vi "String1-2 to OK-NG.vi"(11 "String":string) -> (3 "String Out":string)   [LabVIEW 2021]
doc: "input 1: = OK\ninput 2: = NG\nother \ninput = ouput"
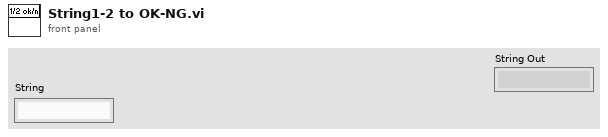
[diagram p1: front panel]
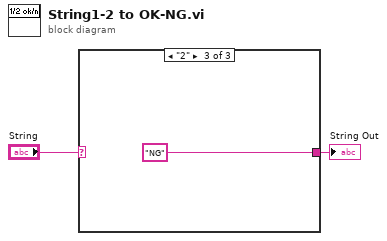
[diagram p0: block diagram]
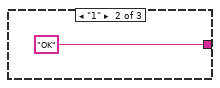
[diagram p3: hidden frame]
diagram:
  n1 = case shown="\"2\"" "String" {
    selector: "String" -> [w3 _ _]
    tunnel: [w3 "OK" "NG"] -> w1
    frame "False", Default {
    }
    frame "1" {
    }
    frame "2" {
    }
  }
  "String Out" <- w1
